vi "Actualizacion Costos.vi"(8 "error in (no error)":errorcluster, 10 "Costo":dbl, 11 "Productos in":refnum<class "Productos.lvclass">) -> (0 "error out":errorcluster, 3 "Productos out":refnum<class "Productos.lvclass">)   [LabVIEW 2020, in "Productos.lvlib" / "Productos.lvclass"]
uses:
  Productos.lvclass
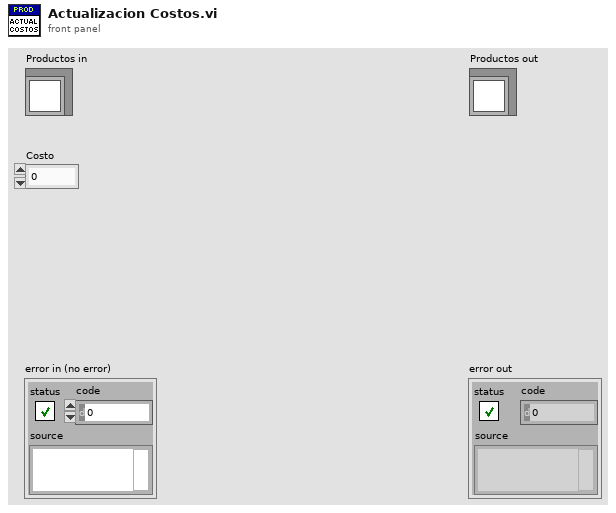
[diagram p1: front panel]
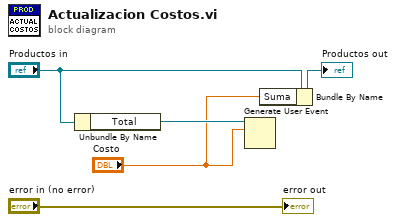
[diagram p0: block diagram]
diagram:
  n1 = Unbundle By Name("Productos in") -> ("Total"=w2:refnum<user-event>)
  n2 = Generate User Event(user event=w2, event data cluster="Costo") -> ()  [unwired: 2 in, 2 out]
  n3 = Bundle By Name(cluster="Productos in", "Suma"="Costo") -> (→"Productos out":refnum<class "Productos.lvclass">)
  "error out" <- "error in (no error)"
